vi "Read Binary Config.vi"(4 "Class Name is Included":bool, 6 "byte order (0:big-endian, network order)":T1(ring), 8 "error in (no error)":errorcluster, 10 "Binary":string, 11 "Const_DBL_1D in":refnum<class "Const_CPLX_DBL_1D.lvclass">) -> (0 "error out":errorcluster, 2 "Remaining":string, 3 "Const_DBL_1D out":refnum<class "Const_CPLX_DBL_1D.lvclass">)   [LabVIEW 2021, in "Const_CPLX_DBL_1D.lvclass"]
uses:
  Const_CPLX_DBL_1D.lvclass
  Const_CPLX_DBL_1D.lvclass/Const_CPLX_DBL_1D.ctl
  Abs_Types/Complex Double Float 1D/Abs_Complex Double Float 1D.lvclass
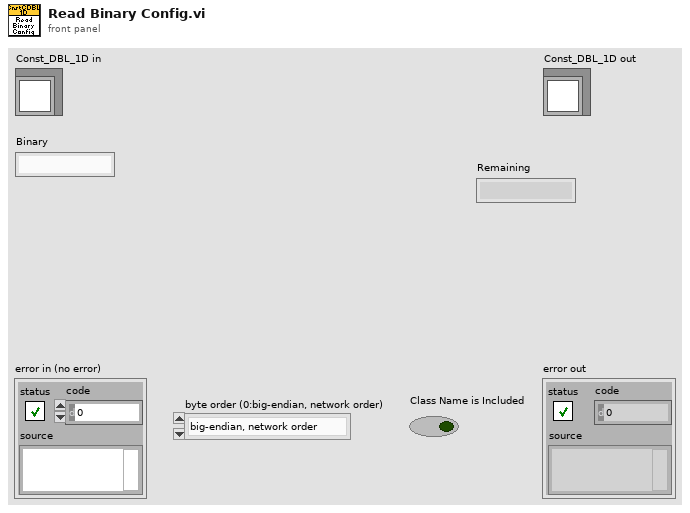
[diagram p1: front panel]
types:
  T1 = enum16{"big-endian, network order", "native, host order", "little-endian"}
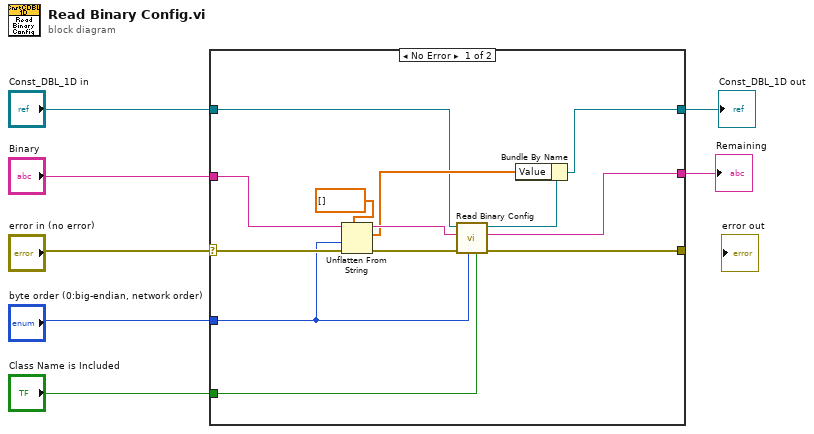
[diagram p0: block diagram]
diagram:
  n1 = case shown="No Error" "error in (no error)" {
    selector: "error in (no error)" -> [w18 w22]
    tunnel: [w13 w22] -> _
    tunnel: [w10 w23] -> w4
    tunnel: "byte order (0:big-endian, network order)" -> [w15 _]
    tunnel: "Const_DBL_1D in" -> [w12 w23]
    tunnel: "Binary" -> [w20 w21]
    tunnel: "Class Name is Included" -> [w9 _]
    tunnel: [w8 w21] -> w3
    frame No Error {
      n2 = Unflatten From String(type=dbl[] [], binary string=w20, byte order (0:big-endian, network order)=w15, error in (no error)=w18) -> (rest of the binary string=w19:string, value=w16:dbl[], error out=w17:errorcluster)  [unwired: 1 in]
      n3 = call-parent "Read Binary Config.vi"("Class Name is Included"=w9, "byte order (0:big-endian, network order)"=w15, "error in (no error)"=w17, "Binary"=w19, "Abs_Type in"=w12) -> ("error out"=w13:errorcluster, "Remaining"=w8:string, "Abs_Type out"=w11:refnum<class "Const_CPLX_DBL_1D.lvclass">)  [unwired: 4 in]
      n4 = Bundle By Name(cluster=w11, "Value"=w16) -> (w10:refnum<class "Const_CPLX_DBL_1D.lvclass">)
    }
    frame Error {
    }
  }
  "Const_DBL_1D out" <- w4
  "Remaining" <- w3
